vi "Scripting_UpdateDerivedClasses.vi"(0 "ClassRef":refnum<vi>, 5 "error in (no error)":errorcluster) -> (19 "error out":errorcluster)   [LabVIEW 2016]
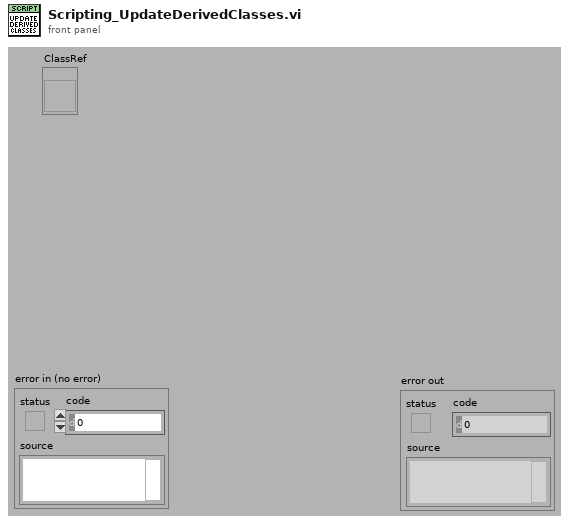
[diagram p1: front panel]
types:
  T1 = cluster{"SubCreate ":path, "RootClassFolder":path, "RootObjectRefPath":path, "AllDerivedClasses":refnum<vi>[], "VIs":refnum<vi>[]}
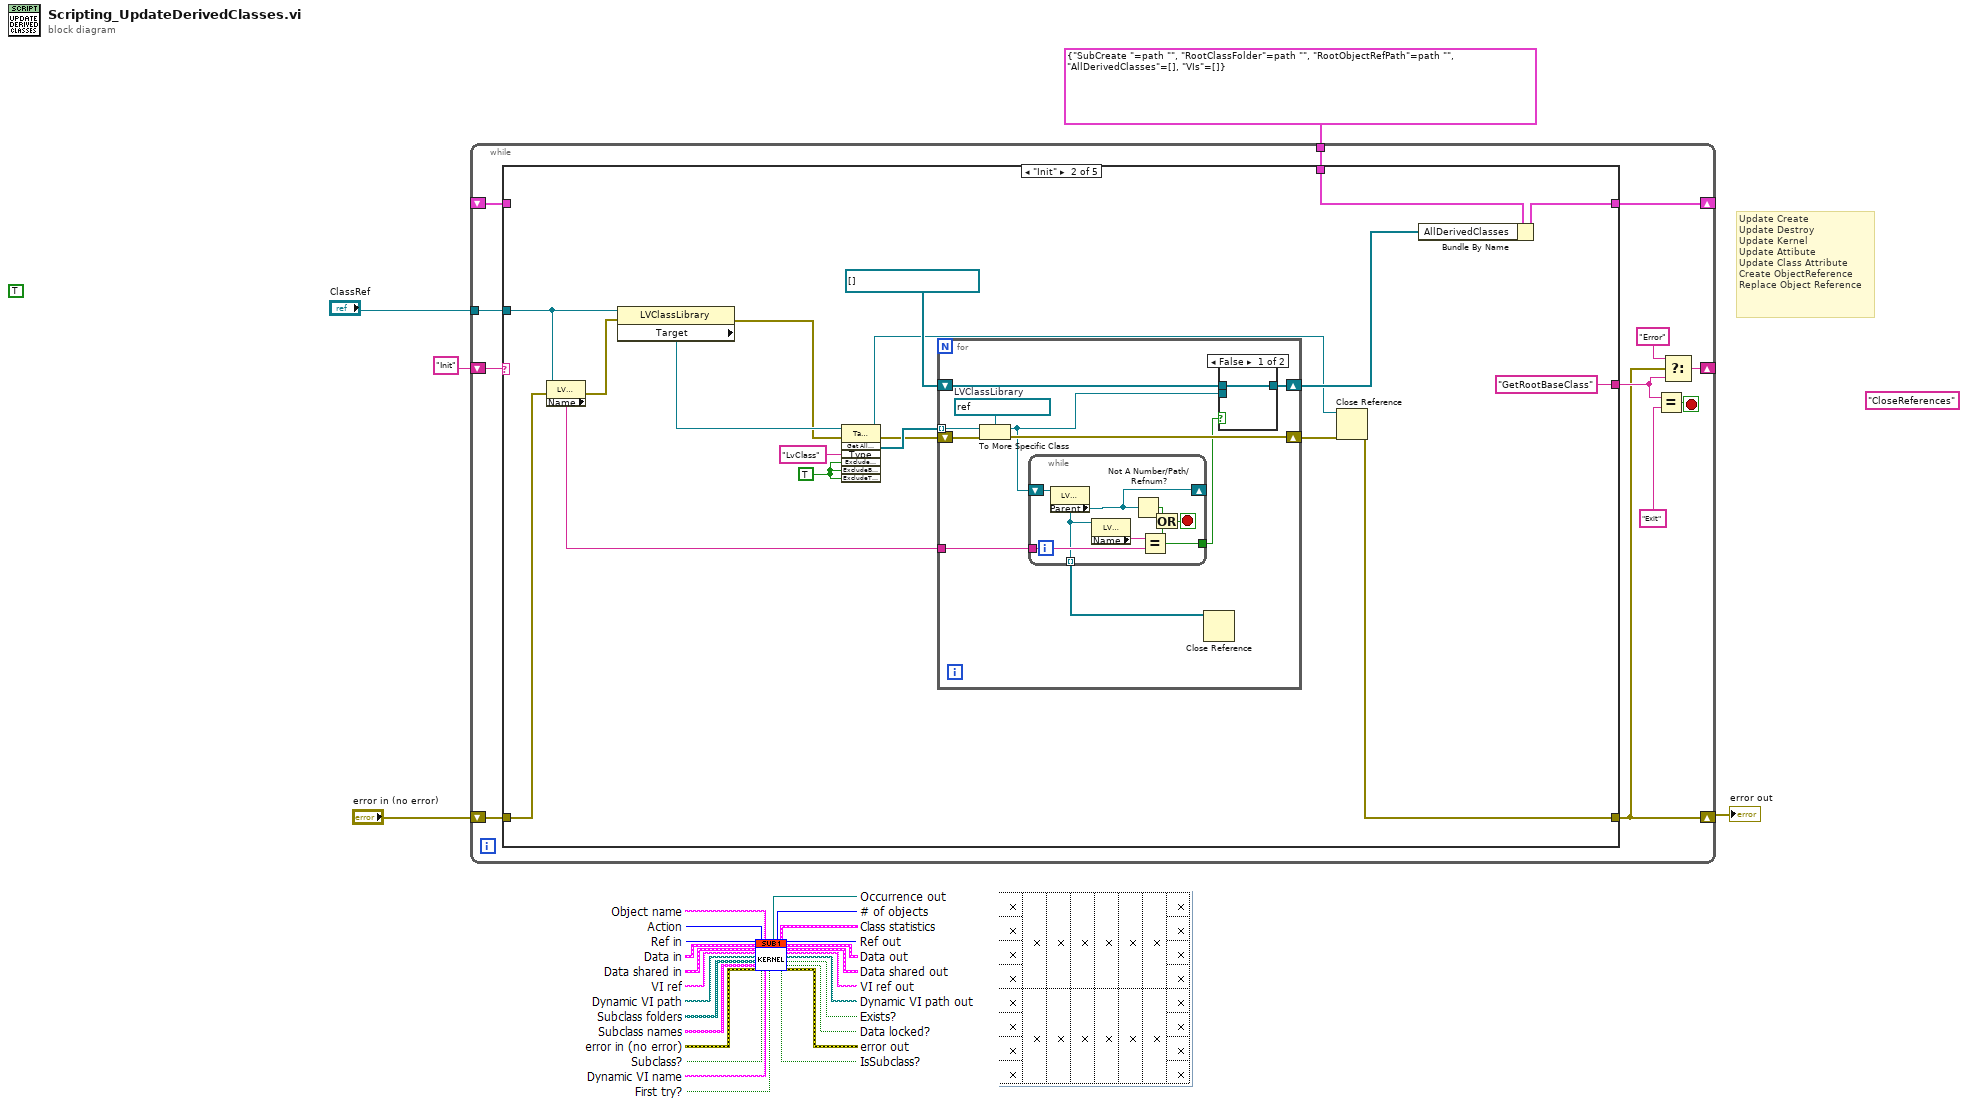
[diagram p0: block diagram]
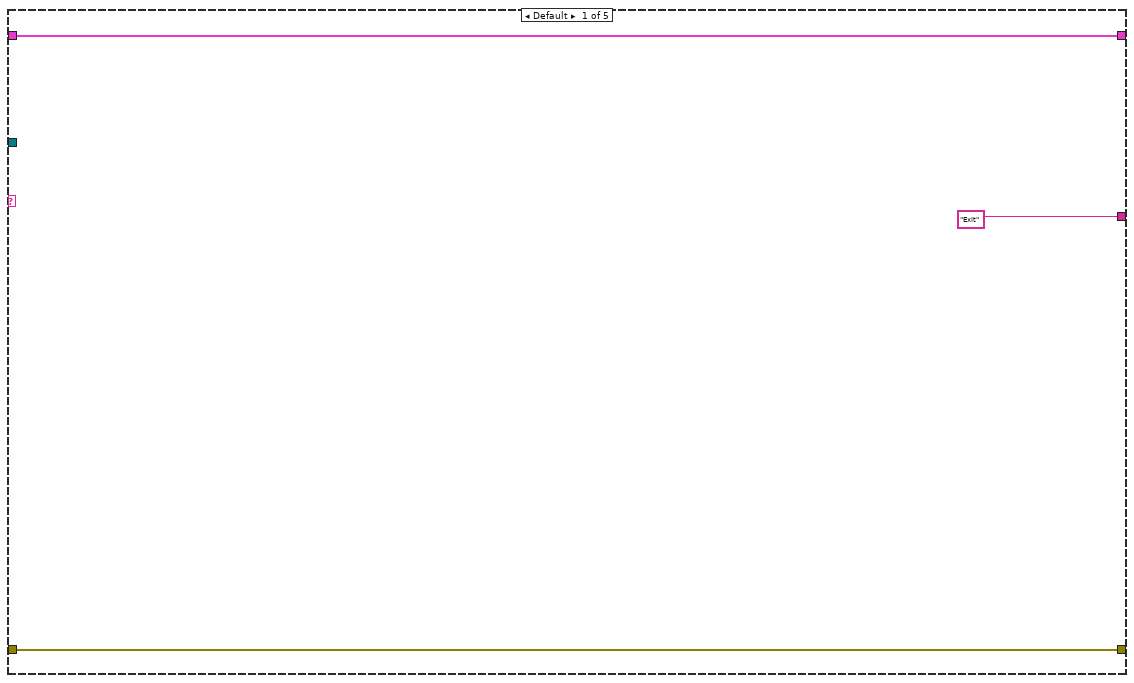
[diagram p2: hidden frame]
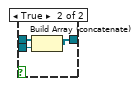
[diagram p3: hidden frame]
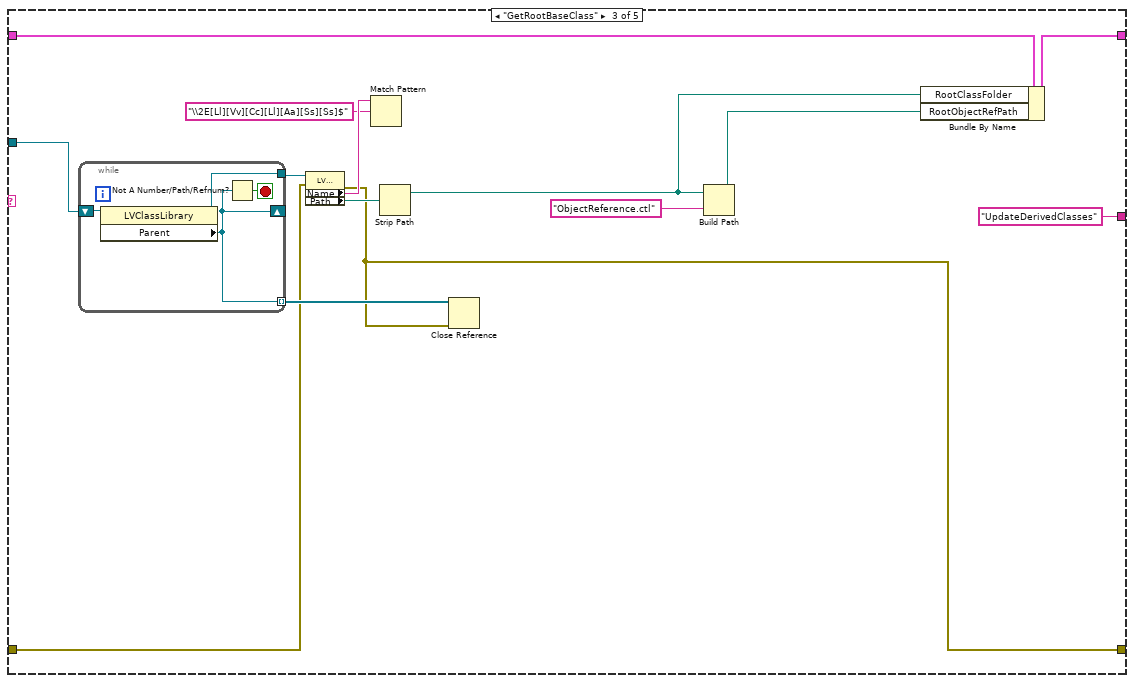
[diagram p4: hidden frame]
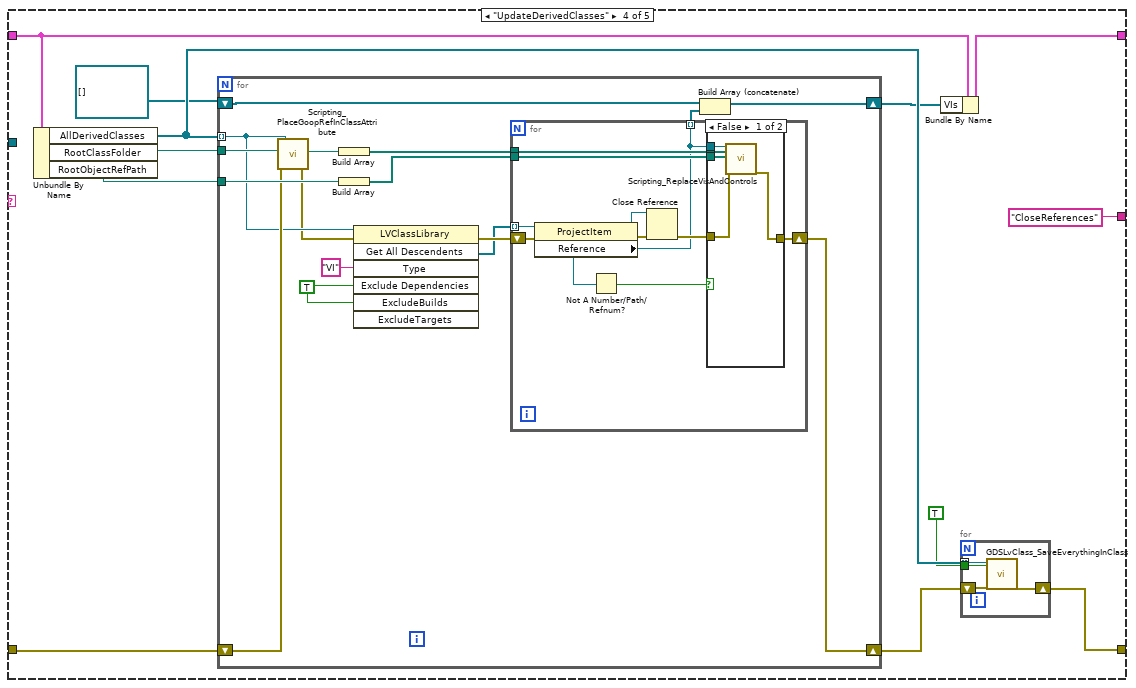
[diagram p5: hidden frame]
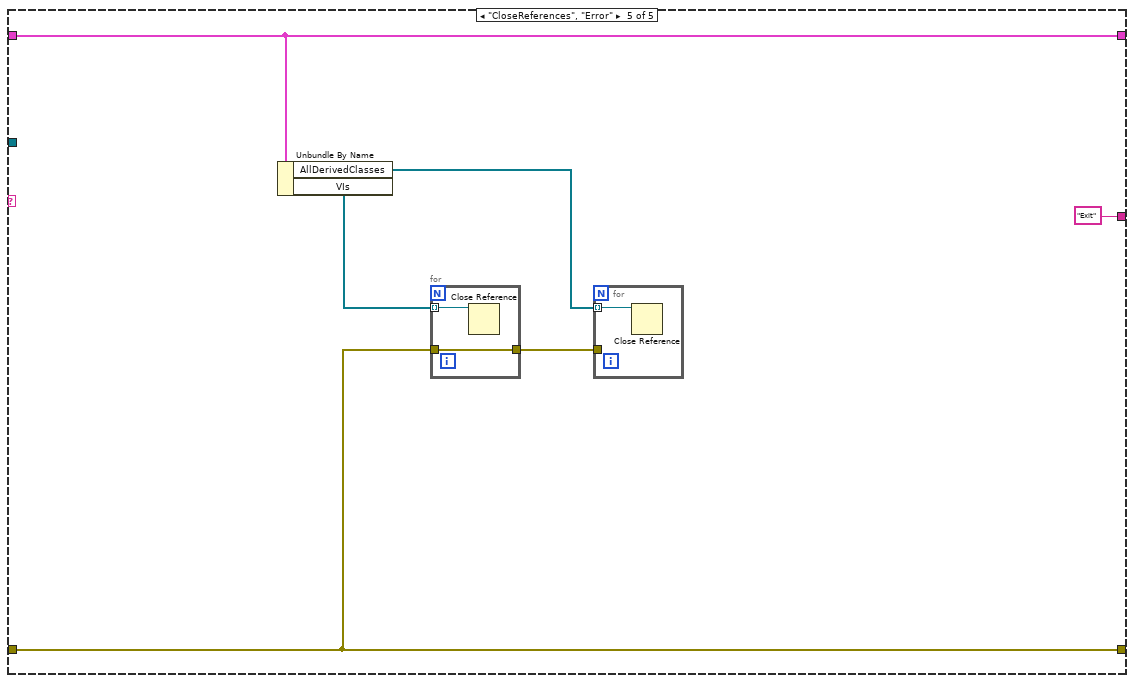
[diagram p7: hidden frame]
diagram:
  (unwired) TRUE
  (unwired) "CloseReferences"
  # "Update Create\nUpdate Destroy\nUpdate Kernel\nUpdate Attibute\nUpdate Class Attribute\nCreate ObjectReference\nReplace Object Reference"
  n1 = while {
    shift-right: [w10] -> w3
    shift-left: "error in (no error)" -> [w17]
    shift-right: [w15] -> _
    shift-left: "Init" -> [w16]
    shift-right: [w9] -> _
    shift-left: _ -> [w8]
    tunnel: "ClassRef" -> [w7]
    tunnel: T1 {"SubCreate "=path "", "RootClassFolder"=path "", "RootObjectRefPath"=path "", "AllDerivedClasses"=[], "VIs"=[]} -> [w6]
    stop <- w14 stop-if-true
    n2 = case shown="\"Init\"" w16 {
      tunnel: w17 -> [w20 w29 w67 w86 w128]
      tunnel: [w20 w22 w60 w84 w128] -> w10
      tunnel: ["Exit" "GetRootBaseClass" "UpdateDerivedClasses" "CloseReferences" "Exit"] -> w11
      tunnel: [w18 w37 w72 w80 w131] -> w9
      tunnel: w8 -> [w18 _ w71 w81 w131]
      tunnel: w7 -> [_ w30 w69 _ _]
      tunnel: w6 -> [_ w36 _ _ _]
      frame Default {
      }
      frame "Init" {
        w34 = TRUE ("ExcludeDependencies")
        n3 = property class="LVClassLibrary"(reference=w30, error in=w29) -> (error out=w28:errorcluster, "Name"=w27:string)  [unwired: 1 out]
        n4 = property class="LVClassLibrary"(reference=w30, error in=w28) -> (error out=w21:errorcluster, "Target"=w23:refnum<vi>)  [unwired: 1 out]
        n5 = invoke class="TargetItem" method="Get All Descendents"(reference=w23, error in=w21, "Type"="LvClass", "Exclude Dependencies"=w34, "ExcludeBuilds"=w34, "ExcludeTargets"=w34) -> (reference out=w24:refnum<vi>, error out=w32:errorcluster, "All Descendents"=w33:refnum<vi>[])  [unwired: 1 in, 4 out]
        n6 = for {
          shift-right: [w47] -> w25
          shift-left: w32 -> [w48]
          tunnel: w33 -> [w46] mode=indexing
          shift-right: [w43] -> w26
          shift-left: refnum<vi>[] [] -> [w44]
          tunnel: w27 -> [w41]
          w45 = refnum<vi> refnum  # LVClassLibrary
          n7 = To More Specific Class(target class=w45, reference=w46, error in=w48) -> (specific class reference=w42:refnum<vi>, error out=w47:errorcluster)
          n8 = while {
            shift-right: [w49] -> _
            shift-left: w42 -> [w55]
            tunnel: w41 -> [w51]
            tunnel: [w50] -> w40
            tunnel: [w49] -> w39 mode=indexing
            stop <- w53 stop-if-true
            n9 = property class="LVClassLibrary"(reference=w55) -> ("Parent"=w49:refnum<vi>)  [unwired: 1 in, 2 out]
            n10 = property class="LVClassLibrary"(reference=w49) -> ("Name"=w52:string)  [unwired: 1 in, 2 out]
            n11 = Not A Number/Path/Refnum?(number/path/refnum=w49) -> (NaN/Path/Refnum?=w54:bool)
            n12 = Equal?(x=w52, y=w51) -> (x = y?=w50:bool)
            n13 = Or(x=w54, y=w50) -> (x .or. y?=w53:bool)
          }
          n14 = Close Reference(reference=w39) -> ()  [unwired: 1 in, 1 out]
          n15 = case shown="False" w40 {
            tunnel: w44 -> [w56 w59]
            tunnel: [w56 w58] -> w43
            tunnel: w42 -> [_ w57]
            frame False {
            }
            frame True {
              n16 = Build Array (concatenate)(w59, w57) -> (w58:refnum<vi>[])
            }
          }
        }
        n17 = Close Reference(reference=w24, error in (no error)=w25) -> (error out=w22:errorcluster)
        n18 = Bundle By Name(cluster=w36, "AllDerivedClasses"=w26) -> (w37:T1)
      }
      frame "GetRootBaseClass" {
        n19 = while {
          shift-right: [w75] -> _
          shift-left: w69 -> [w76]
          tunnel: [w75] -> w70 mode=indexing
          tunnel: [w74] -> w68
          stop <- w77 stop-if-true
          n20 = property class="LVClassLibrary"(reference=w76) -> (reference out=w74:refnum<vi>, "Parent"=w75:refnum<vi>)  [unwired: 1 in, 1 out]
          n21 = Not A Number/Path/Refnum?(number/path/refnum=w75) -> (NaN/Path/Refnum?=w77:bool)
        }
        n22 = property class="LVClassLibrary"(reference=w68, error in=w67) -> (error out=w60:errorcluster, "Name"=w66:string, "Path"=w64:path)  [unwired: 1 out]
        n23 = Match Pattern(string=w66, regular expression="\\2E[Ll][Vv][Cc][Ll][Aa][Ss][Ss]$") -> ()  [unwired: 1 in, 4 out]
        n24 = Strip Path(path=w64) -> (stripped path=w62:path)  [unwired: 1 out]
        n25 = Close Reference(reference=w70, error in (no error)=w60) -> ()  [unwired: 1 out]
        n26 = Build Path(base path=w62, name or relative path="ObjectReference.ctl" ("element")) -> (appended path=w63:path)
        n27 = Bundle By Name(cluster=w71, "RootClassFolder"=w62, "RootObjectRefPath"=w63) -> (w72:T1)
      }
      frame "UpdateDerivedClasses" {
        n28 = Unbundle By Name(w81) -> ("AllDerivedClasses"=w83:refnum<vi>[], "RootClassFolder"=w88:path, "RootObjectRefPath"=w87:path)
        n29 = for {
          tunnel: w88 -> [w109]
          tunnel: w87 -> [w106]
          shift-right: [w103] -> w85
          shift-left: w86 -> [w104]
          tunnel: w83 -> [w100] mode=indexing
          shift-right: [w101] -> w79
          shift-left: refnum<vi>[] [] -> [w102]
          w94 = TRUE ("ExcludeDependencies")
          n30 = call <resource>:"Scripting_PlaceGoopRefInClassAttribute.vi"("error in"=w104, "ObjectRef_LvClassFolderPath"=w109, "ClassRefnum"=w100) -> ("error out"=w99:errorcluster, "ReplacedObjectRef(ifOldRefFound)"=w108:path)  [unwired: 1 in, 2 out]
          n31 = Build Array(w108) -> (w107:path[])
          n32 = Build Array(w106) -> (w105:path[])
          n33 = invoke class="LVClassLibrary" method="Get All Descendents"(reference=w100, error in=w99, "Type"="VI", "Exclude Dependencies"=w94, "ExcludeBuilds"=w94) -> (error out=w98:errorcluster, "All Descendents"=w97:refnum<vi>[])  [unwired: 2 in, 5 out]
          n34 = for {
            shift-right: [w119] -> w103
            shift-left: w98 -> [w116]
            tunnel: w107 -> [w118]
            tunnel: w105 -> [w117]
            tunnel: w97 -> [w115] mode=indexing
            tunnel: [w110] -> w95 mode=indexing
            n35 = property class="ProjectItem"(reference=w115, error in=w116) -> (reference out=w113:refnum<vi>, error out=w114:errorcluster, "Reference"=w110:refnum<vi>)
            n36 = Not A Number/Path/Refnum?(number/path/refnum=w110) -> (NaN/Path/Refnum?=w112:bool)
            n37 = Close Reference(reference=w113, error in (no error)=w114) -> (error out=w111:errorcluster)
            n38 = case shown="False" w112 {
              tunnel: [w124 w125] -> w119
              tunnel: w118 -> [w123 _]
              tunnel: w117 -> [w122 _]
              tunnel: w111 -> [w121 w125]
              tunnel: w110 -> [w120 _]
              frame False {
                n39 = call <resource>:"Scripting_ReplaceVisAndControls.vi"("ViRef"=w120, "OldVIsAndControls"=w123, "NewVIsAndControls"=w122, "error in (no error)"=w121) -> ("error out"=w124:errorcluster)  [unwired: 14 in, 1 out]
              }
              frame True {
              }
            }
          }
          n40 = Build Array (concatenate)(w102, w95) -> (w101:refnum<vi>[])
        }
        n41 = Bundle By Name(cluster=w81, "VIs"=w79) -> (w80:T1)
        n42 = for {
          tunnel: w83 -> [w91] mode=indexing
          shift-right: [w93] -> w84
          shift-left: w85 -> [w92]
          tunnel: TRUE ("ForceResaving(False)") -> [w90]
          n43 = call <resource>:"GDSLvClass_SaveEverythingInClass.vi"("ClassRefIn"=w91, "ForceResaving(False)"=w90, "error in"=w92) -> ("error out"=w93:errorcluster)  [unwired: 15 in, 1 out]
        }
      }
      frame "CloseReferences", "Error" {
        n44 = Unbundle By Name(w131) -> ("AllDerivedClasses"=w129:refnum<vi>[], "VIs"=w126:refnum<vi>[])
        n45 = for {
          tunnel: w126 -> [w133] mode=indexing
          tunnel: w128 -> [w132]
          tunnel: [w132] -> w127
          n46 = Close Reference(reference=w133) -> ()  [unwired: 1 in, 1 out]
        }
        n47 = for {
          tunnel: w129 -> [w134] mode=indexing
          tunnel: w127 -> [_]
          n48 = Close Reference(reference=w134) -> ()  [unwired: 1 in, 1 out]
        }
      }
    }
    n49 = Equal?(x=w11, y="Exit") -> (x = y?=w14:bool)
    n50 = Select(t="Error", s=w10, f=w11) -> (s? t:f=w15:string)
  }
  "error out" <- w3
